vi "Task.vi"() -> ()   [LabVIEW 2019]
panel:
  out "Boolean":bool
  out "Numeric 2":dbl
  out "Tank 2":dbl(slide) scale=0.0..10.0
  out "Numeric":dbl
  out "Tank":dbl(slide) scale=0.0..10.0
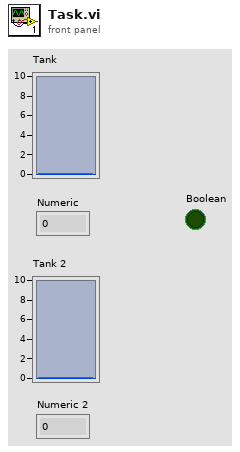
[diagram p1: front panel]
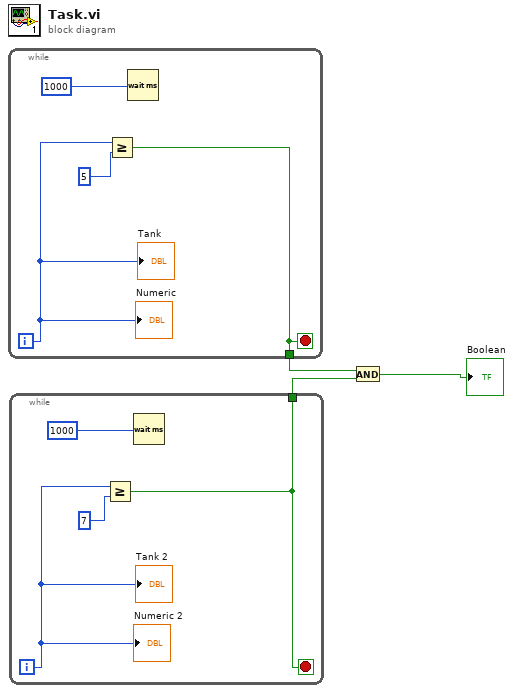
[diagram p0: block diagram]
diagram:
  n1 = while {
    tunnel: [w4] -> w2
    i -> [w5]
    stop <- w4 stop-if-true
    n2 = Greater Or Equal?(x=w5, y=5) -> (x >= y?=w4:bool)
    n3 = Wait (ms)(milliseconds to wait=1000) -> ()  [unwired: 1 out]
    "Tank" <- w5
    "Numeric" <- w5
  }
  n4 = while {
    tunnel: [w8] -> w3
    i -> [w9]
    stop <- w8 stop-if-true
    n5 = Greater Or Equal?(x=w9, y=7) -> (x >= y?=w8:bool)
    n6 = Wait (ms)(milliseconds to wait=1000) -> ()  [unwired: 1 out]
    "Tank 2" <- w9
    "Numeric 2" <- w9
  }
  n7 = And(x=w2, y=w3) -> (x .and. y?=→"Boolean":bool)
